vi "RYB Complementary Color.vi"(11 "Color in":u32(colorbox)=16744448) -> (3 "Complementary Color":u32(colorbox)=16744448)   [LabVIEW 2015, in "ColorSelector.lvclass"]
doc: "This VI determines the Complementary Color of the input color in the RYB Color Scale.\n<b> </b> <b> </b>\n©2017 Q Software Innovations, LLC (QSI)\nwritten by Quentin Alldredge\nproduced in LabVIEW 2015\n\nsupport@qsoftwareinnovations.com\nwww.qsoftwareinnovations.com\n\nAll rights reserved.\n\nRedistribution and use in source and binary forms, with or without modification, are permitted provided that the following conditions are met:\n\n * Redistributions of source code must retain the above copyright notice, this list of conditions and the following disclaimer.\n * Redistributions in binary form must reproduce the above copyright notice, this list of conditions and the following disclaimer in the documentation and/or other materials provided with the distribution.\n * Neither the name of Q Software Innovations, LLC. nor the names of its contributors may be used to endorse or promote products derived from this software without specific prior written permission.\n\nTHIS SOFTWARE IS PROVIDED BY THE COPYRIGHT HOLDERS AND CONTRIBUTORS \"AS IS\" AND ANY EXPRESS OR IMPLIED WARRANTIES, INCLUDING, BUT NOT LIMITED TO, THE IMPLIED WARRANTIES OF MERCHANTABILITY AND FITNESS FOR A PARTICULAR PURPOSE ARE DISCLAIMED. IN NO EVENT SHALL THE COPYRIGHT OWNER OR CONTRIBUTORS BE LIABLE FOR ANY DIRECT, INDIRECT, INCIDENTAL, SPECIAL, EXEMPLARY, OR CONSEQUENTIAL DAMAGES (INCLUDING, BUT NOT LIMITED TO, PROCUREMENT OF SUBSTITUTE GOODS OR SERVICES; LOSS OF USE, DATA, OR PROFITS; OR BUSINESS INTERRUPTION) HOWEVER CAUSED AND ON ANY THEORY OF LIABILITY, WHETHER IN CONTRACT, STRICT LIABILITY, OR TORT (INCLUDING NEGLIGENCE OR OTHERWISE) ARISING IN ANY WAY OUT OF THE USE OF THIS SOFTWARE, EVEN IF ADVISED OF THE POSSIBILITY OF SUCH DAMAGE."
uses:
  ColorSelector.lvclass
panel:
  out "error out (dup)":errorcluster
  in  "error in (no error)":errorcluster
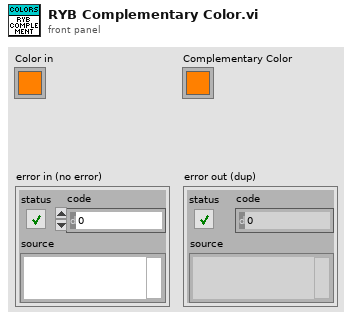
[diagram p1: front panel]
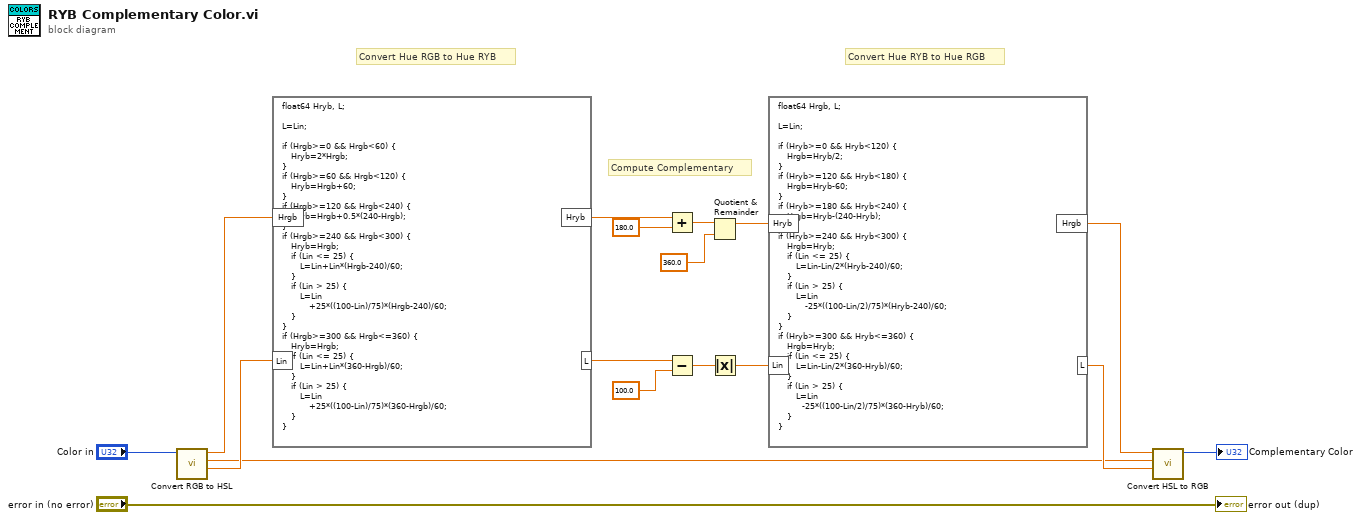
[diagram p0: block diagram]
diagram:
  # "Compute Complementary"
  # "Convert Hue RYB to Hue RGB"
  # "Convert Hue RGB to Hue RYB"
  n1 = call "Convert RGB to HSL.vi"("Color Box"="Color in") -> ("L (%)"=w3:dbl, "S (%)"=w1:dbl, "H (deg)"=w15:dbl)  [unwired: 8 in]
  n2 = formula code="float64 Hryb, L;\n\nL=Lin;\n\nif (Hrgb>=0 && Hrgb<60) {\n   Hryb=2*Hrgb;\n}\nif (Hrgb>=60 && Hrgb<120) {\n   Hryb=Hrgb+60;\n}\nif (Hrgb>=120 && Hrgb<240) {\n   Hryb=Hrgb+0.5*(240-Hrgb);\n}\nif (Hrgb>=240 && Hrgb<300) {\n   Hryb=Hrgb;\n   if (Lin <= 25) {\n      L=Lin+Lin*(Hrgb-240)/60;\n   }\n   if (Lin > 25) {\n      L=Lin\n         +25*((100-Lin)/75)*(Hrgb-240)/60;\n   }\n}\nif (Hrgb>=300 && Hrgb<=360) {\n   Hryb=Hrgb;\n   if (Lin <= 25) {\n      L=Lin+Lin*(360-Hrgb)/60;\n   }\n   if (Lin > 25) {\n      L=Lin\n         +25*((100-Lin)/75)*(360-Hrgb)/60;\n   }\n}"("Hrgb"=w15, "Lin"=w3) -> ("Hryb"=w13:dbl, "L"=w7:dbl)
  n3 = Add(x=w13, y=180.0) -> (x+y=w11:dbl)
  n4 = Subtract(x=w7, y=100.0) -> (x-y=w5:dbl)
  n5 = Quotient & Remainder(x=w11, y=360.0) -> (x-y*floor(x/y)=w8:dbl)  [unwired: 1 out]
  n6 = Absolute Value(x=w5) -> (abs(x)=w4:dbl)
  n7 = formula code="float64 Hrgb, L;\n\nL=Lin;\n\nif (Hryb>=0 && Hryb<120) {\n   Hrgb=Hryb/2;\n}\nif (Hryb>=120 && Hryb<180) {\n   Hrgb=Hryb-60;\n}\nif (Hryb>=180 && Hryb<240) {\n   Hrgb=Hryb-(240-Hryb);\n}\nif (Hryb>=240 && Hryb<300) {\n   Hrgb=Hryb;\n   if (Lin <= 25) {\n      L=Lin-Lin/2*(Hryb-240)/60;\n   }\n   if (Lin > 25) {\n      L=Lin\n         -25*((100-Lin/2)/75)*(Hryb-240)/60;\n   }\n}\nif (Hryb>=300 && Hryb<=360) {\n   Hrgb=Hryb;\n   if (Lin <= 25) {\n      L=Lin-Lin/2*(360-Hryb)/60;\n   }\n   if (Lin > 25) {\n      L=Lin\n        -25*((100-Lin/2)/75)*(360-Hryb)/60;\n   }\n}"("Hryb"=w8, "Lin"=w4) -> ("Hrgb"=w9:dbl, "L"=w2:dbl)
  n8 = call "Convert HSL to RGB.vi"("L (%)"=w2, "S (%)"=w1, "H (deg)"=w9) -> ("Color Box"=→"Complementary Color":u32)  [unwired: 8 in]
  "error out (dup)" <- "error in (no error)"
